vi "tankstatus.vi"(7 "LabVIEW Web Service Request":refnum<class "Web Request.lvclass">) -> ()   [LabVIEW 2019]
uses:
  <vilib>/wsapi/Web Request.lvclass
panel:
  # "Use the Web Service Request input terminal to call the VIs on the Web Services palette. Do not remove it from the connector pane unless you don't need access to the palette."
  # "Each additional control wired to the connector pane will be available as an input in the URL. To include an indicator in terminal-mode output (the default setting), it must also be wired to the connector pane."
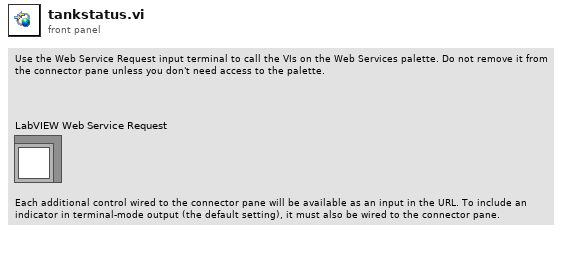
[diagram p1: front panel]
types:
  T1 = typedef "JSON_Tank.ctl" = cluster{"number":u16, "building":string, "room":string, "ipAddress":string, "profileName":string, "caNumber":string, "ctrlType":string, "mode":string, "channels":T2[], "pumps":T3[]}
  T2 = typedef "JSON_Channel.ctl" = cluster{"name":string, "tag":string, "data":string, "type":string, "unit":string}
  T3 = typedef "JSON_Pump.ctl" = cluster{"position":u8, "enabled":bool, "command":string, "channels":T2[], "elapsedTime":string}
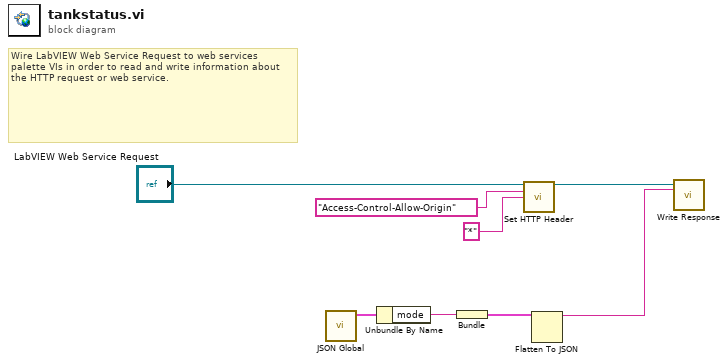
[diagram p0: block diagram]
diagram:
  # "Wire LabVIEW Web Service Request to web services palette VIs in order to read and write information about the HTTP request or web service."
  n1 = call "JSON Global.vi"() -> ("JSON Out"=w3:T1)  [unwired: 11 in]
  n2 = Unbundle By Name(w3) -> ("mode"=w2:string)
  n3 = Bundle("mode"=w2) -> (w1:cluster{"mode":string})  [unwired: 1 in]
  n4 = call <vilib>:"Set HTTP Header.vi"("LabVIEW Web Service Request"="LabVIEW Web Service Request", "header"="Access-Control-Allow-Origin" ("header value"), "header value"="*" ("header")) -> ("LabVIEW Web Service Request out"=w7:refnum<class "Web Request.lvclass">)  [unwired: 11 in, 1 out]
  n5 = Flatten To JSON(anything=w1) -> (JSON string=w4:string)  [unwired: 2 in, 1 out]
  n6 = call <vilib>:"Write Response.vi"("LabVIEW Web Service Request"=w7, "response string"=w4) -> ()  [unwired: 12 in, 2 out]
